vi "Order check.vi"(11 "Wire in in":T1) -> (3 "Wire out":T1)   [LabVIEW 2016]
uses:
  TypeDefs/Circuit Cluster.ctl
  Classes/GateAbst/GateAbst.lvclass
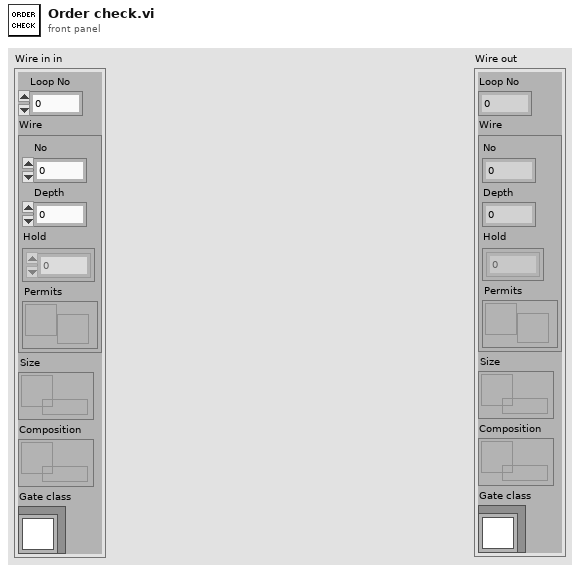
[diagram p1: front panel]
types:
  T1 = typedef "Circuit Cluster.ctl" = cluster{"Loop No":i32, "Wire":cluster{"No":i32, "Depth":i32, "Hold":i32[][], "Permits":refnum<notifier>}, "Size":refnum<queue>, "Composition":refnum<queue>, "Gate class":refnum<class "GateAbst.lvclass">}
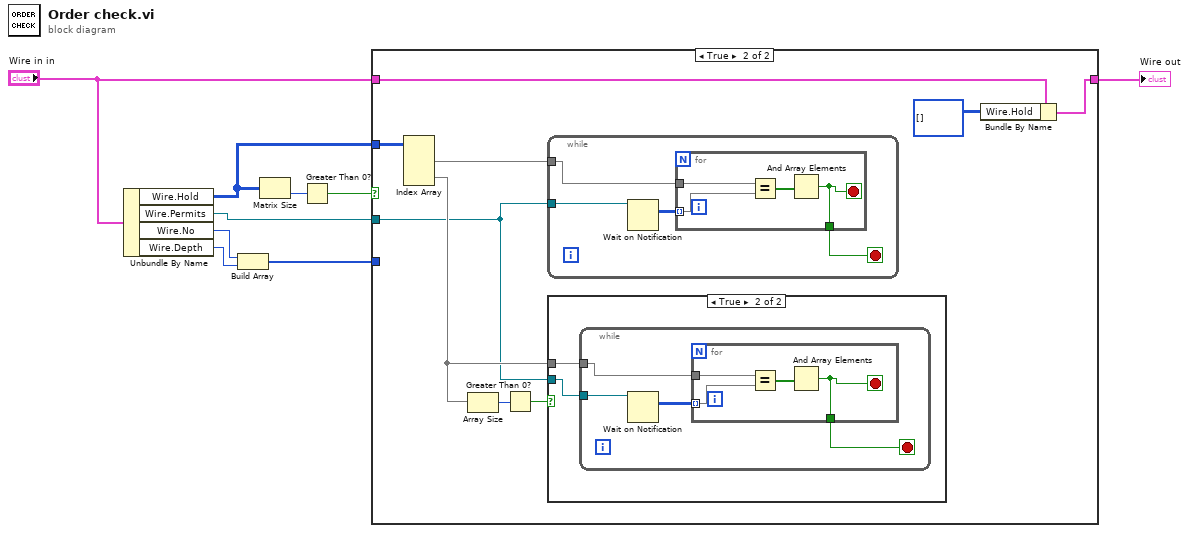
[diagram p0: block diagram]
diagram:
  n1 = Unbundle By Name("Wire in in") -> ("Wire.Hold"=w2:i32[][], "Wire.Permits"=w1:refnum<notifier>, "Wire.No"=w5:i32, "Wire.Depth"=w6:i32)
  n2 = Build Array(w5, w6) -> (w7:i32[])
  n3 = Matrix Size(0:w2) -> (2:w3:i32)  [unwired: 1 out]
  n4 = Greater Than 0?(x=w3) -> (x > 0?=w4:bool)
  n5 = case shown="True" w4 {
    tunnel: w7 -> [_ _]
    tunnel: "Wire in in" -> [w10 w19]
    tunnel: [w10 w18] -> w9
    tunnel: w2 -> [_ w16]
    tunnel: w1 -> [_ w11]
    frame False {
    }
    frame True {
      n6 = Index Array(array=w16) -> (element #1=w15:i32[], element #2=w12:i32[])  [unwired: 4 in]
      n7 = Array Size(array=w12) -> (size(s)=w13:i32)
      n8 = Greater Than 0?(x=w13) -> (x > 0?=w14:bool)
      n9 = while {
        tunnel: w11 -> [w31]
        tunnel: w15 -> [w32]
        stop <- w33 stop-if-true
        n10 = Wait on Notification(notifier=w31) -> (notification=w30:i32[][])  [unwired: 3 in, 3 out]
        n11 = for {
          tunnel: [w34] -> w33
          tunnel: w32 -> [w37]
          tunnel: w30 -> [w35] mode=indexing
          stop <- w34 stop-if-true
          n12 = Equal?(x=w37, y=w35) -> (x = y?=w36:bool[])
          n13 = And Array Elements(Boolean array=w36) -> (logical AND=w34:bool)
        }
      }
      n14 = case shown="True" w14 {
        tunnel: w11 -> [_ w20]
        tunnel: w12 -> [_ w21]
        frame False {
        }
        frame True {
          n15 = while {
            tunnel: w20 -> [w23]
            tunnel: w21 -> [w24]
            stop <- w25 stop-if-true
            n16 = Wait on Notification(notifier=w23) -> (notification=w22:i32[][])  [unwired: 3 in, 3 out]
            n17 = for {
              tunnel: [w26] -> w25
              tunnel: w24 -> [w29]
              tunnel: w22 -> [w27] mode=indexing
              stop <- w26 stop-if-true
              n18 = Equal?(x=w29, y=w27) -> (x = y?=w28:bool[])
              n19 = And Array Elements(Boolean array=w28) -> (logical AND=w26:bool)
            }
          }
        }
      }
      n20 = Bundle By Name(cluster=w19, "Wire.Hold"=i32[][] []) -> (w18:T1)
    }
  }
  "Wire out" <- w9
